vi "Передать кластер параметров в TCP (SubVI).vi"(7 "Кластер параметров мишени":T1, 11 "error in":errorcluster, 13 "TCP connection ID":refnum<k5>) -> (8 "bytes written to TCP":i32, 15 "error out":errorcluster)   [LabVIEW 2015]
doc: "Передача всех параметров мишеней в МК по TCP"
panel:
  out "string":string
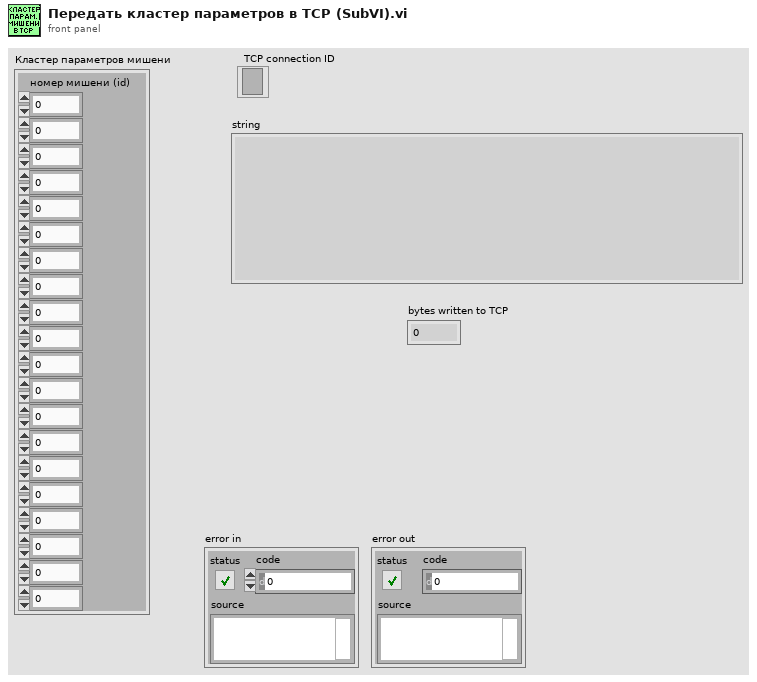
[diagram p1: front panel]
types:
  T1 = cluster{"номер мишени (id)":u8, u8, u8, u8, u8, u8, u8, u8, u8, u8, u8, u8, u8, u8, u8, u8, u8, u8, u8, u8}
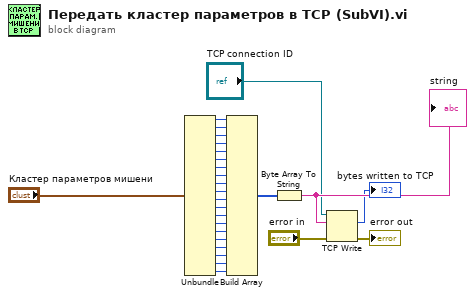
[diagram p0: block diagram]
diagram:
  n1 = Unbundle("Кластер параметров мишени") -> ("номер мишени (id)"=w7:u8, w8:u8, w9:u8, w10:u8, w11:u8, w12:u8, w13:u8, w14:u8, w15:u8, w16:u8, w17:u8, w18:u8, w19:u8, w20:u8, w21:u8, w22:u8, w23:u8, w24:u8, w25:u8, w26:u8)
  n2 = Build Array(w7, w8, w9, w10, w11, w12, w13, w14, w15, w16, w17, w18, w19, w20, w21, w22, w23, w24, w25, w26) -> (w27:u8[])
  n3 = Byte Array To String(unsigned byte array=w27) -> (string=w5:string)
  "string" <- w5
  n4 = TCP Write(connection ID="TCP connection ID", data in=w5, error in (no error)="error in") -> (bytes written=→"bytes written to TCP":i32, error out=→"error out":errorcluster)  [unwired: 1 in, 1 out]
